vi "BallPossession.vi"(10 "IA State Input":T1) -> (2 "Posse inimigo":bool)   [LabVIEW 2016]
uses:
  Core/AI Input.ctl
  Core/AI Robot.ctl
  Intel/Functions Enum.ctl
  Core/AI Ball.ctl
  Core/Field Size.ctl
  Core/AI Judge.ctl
  Intel/Command Enum.ctl
  <vilib>/Analysis/coordinate.llb/Wrap Angle (scalar).vi
  <vilib>/Analysis/NI_AAL_Angle.lvlib
panel:
  in  "Tol para ang posse":dbl=0.3
  in  "Dist Para posse":dbl=180.0
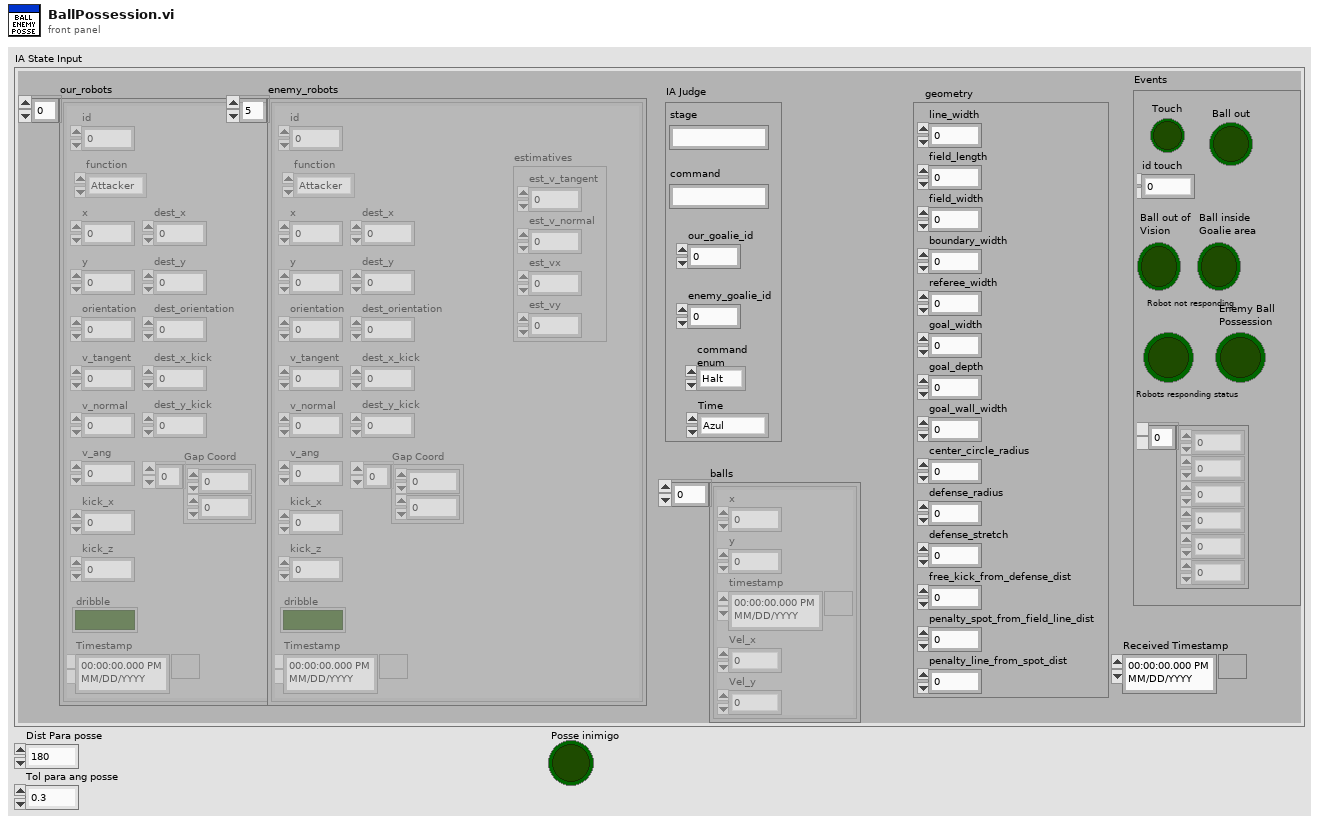
[diagram p1: front panel]
types:
  T1 = typedef "AI Input.ctl" = cluster{"our_robots":T2[], "enemy_robots":T2[], "balls":T4[], "geometry":T5, "IA Judge":T6, "Received Timestamp":timestamp, "Events":cluster{"Touch":bool, "Ball out":bool, "id touch":dbl, "Ball out of \nVision":bool, "Ball inside \nGoalie area":bool, "Robot not responding":bool, "Robots responding status":dbl[], "Enemy Ball \nPossession":bool}}
  T2 = typedef "AI Robot.ctl" = cluster{"id":u32, "function":T3, "x":dbl, "y":dbl, "orientation":dbl, "v_tangent":dbl, "v_normal":dbl, "v_ang":dbl, "kick_x":dbl, "kick_z":dbl, "dribble":bool, "Timestamp":timestamp, "dest_x":dbl, "dest_y":dbl, "dest_orientation":dbl, "estimatives":cluster{"est_v_tangent":dbl, "est_v_normal":dbl, "est_vx":dbl, "est_vy":dbl}, "dest_x_kick":dbl, "dest_y_kick":dbl, "Gap Coord":dbl[]}
  T3 = typedef "Functions Enum.ctl" = enum16{"Attacker", "Goalie", "Defender", "Striker", "Goto 0", "Dummy", "Kicker", "ZigZag"}
  T4 = typedef "AI Ball.ctl" = cluster{"x":dbl, "y":dbl, "timestamp":timestamp, "Vel_x":dbl, "Vel_y":dbl}
  T5 = typedef "Field Size.ctl" = cluster{"line_width":u32, "field_length":u32, "field_width":u32, "boundary_width":u32, "referee_width":u32, "goal_width":u32, "goal_depth":u32, "goal_wall_width":u32, "center_circle_radius":u32, "defense_radius":u32, "defense_stretch":u32, "free_kick_from_defense_dist":u32, "penalty_spot_from_field_line_dist":u32, "penalty_line_from_spot_dist":u32}
  T6 = typedef "AI Judge.ctl" = cluster{"stage":string, "command":string, "our_goalie_id":dbl, "enemy_goalie_id":dbl, "command\nenum":T7, "Time":enum16{"Azul", "Amarelo"}}
  T7 = typedef "Command Enum.ctl" = enum16{"Halt", "Stop", "Force Start", "PKA Normal Start", "Prepare Kickoff Ally", "PKE Normal Start", "Prepare Kickoff Enemy", "Prepare Penalty Ally", "PPA Normal Start", "Prepare Penalty Enemy", "PPE Normal Start", "Direct Free Enemy", "Direct Free Ally", "Indirect Free Enemy", "Indirect Free Ally", "Timeout Enemy", "Timeout Ally", "Goal Enemy", "Goal Ally", "Ball Placement Enemy", "Ball Placement Ally", "None"}
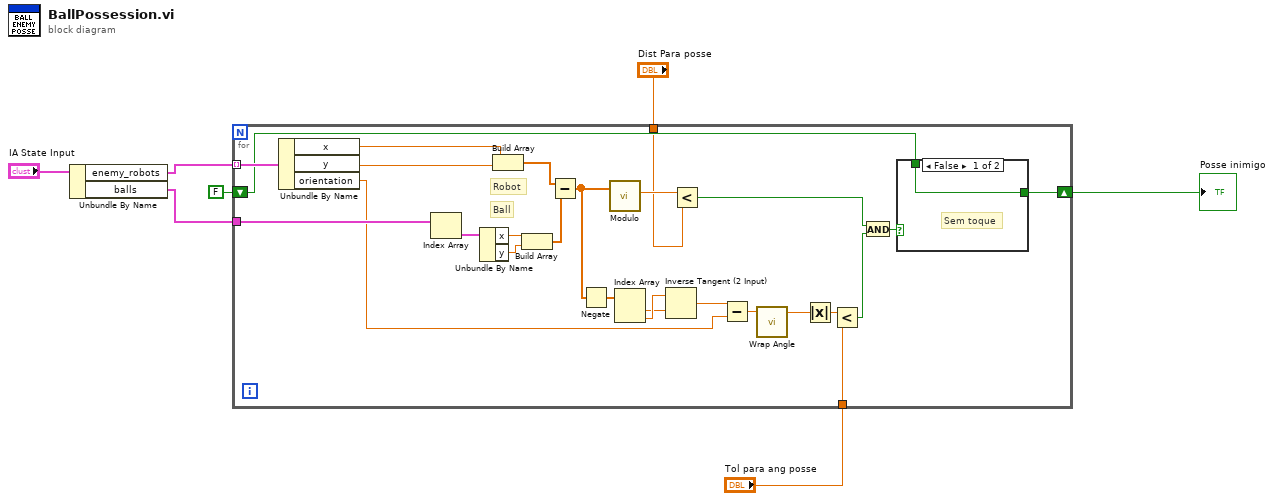
[diagram p0: block diagram]
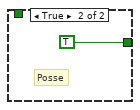
[diagram p2: hidden frame]
diagram:
  n1 = Unbundle By Name("IA State Input") -> ("enemy_robots"=w6:T2[], "balls"=w5:T4[])
  n2 = for {
    tunnel: w6 -> [w29] mode=indexing
    tunnel: w5 -> [w33]
    shift-right: [w23] -> w2
    shift-left: FALSE -> [w22]
    tunnel: "Dist Para posse" -> [w21]
    tunnel: "Tol para ang posse" -> [w14]
    # "Ball"
    # "Robot"
    n3 = Unbundle By Name(w29) -> ("x"=w28:dbl, "y"=w27:dbl, "orientation"=w15:dbl)
    n4 = Index Array(array=w33) -> (element=w32:T4)  [unwired: 1 in]
    n5 = Unbundle By Name(w32) -> ("x"=w31:dbl, "y"=w30:dbl)
    n6 = Build Array(w28, w27) -> (w26:dbl[])
    n7 = Build Array(w31, w30) -> (w25:dbl[])
    n8 = Subtract(x=w26, y=w25) -> (x-y=w20:dbl[])
    n9 = Negate(x=w20) -> (-x=w19:dbl[])
    n10 = call "Modulo.vi"("2D vector"=w20) -> ("Modulo"=w24:dbl)  [unwired: 10 in]
    n11 = Index Array(array=w19) -> (element #1=w17:dbl, element #2=w18:dbl)  [unwired: 2 in]
    n12 = Inverse Tangent (2 Input)(1:w17, 2:w18) -> (0:w16:dbl)
    n13 = Less?(x=w24, y=w21) -> (x < y?=w12:bool)
    n14 = Subtract(x=w16, y=w15) -> (x-y=w10:dbl)
    n15 = call-poly <vilib>:"Wrap Angle.vi"("angle in"=w10) -> ("angle out"=w8:dbl)  [unwired: 9 in, 1 out]
    n16 = Absolute Value(x=w8) -> (abs(x)=w9:dbl)
    n17 = Less?(x=w9, y=w14) -> (x < y?=w13:bool)
    n18 = And(x=w12, y=w13) -> (x .and. y?=w11:bool)
    n19 = case shown="False" w11 {
      tunnel: [w34 TRUE] -> w23
      tunnel: w22 -> [w34 _]
      frame False {
        # "Sem toque"
      }
      frame True {
        # "Posse"
      }
    }
  }
  "Posse inimigo" <- w2
